vi "Auto_Routine_RightTwoPieceThen2CenterTRAJ.vi"   [LabVIEW 2023]
uses:
  Shoulder/ShoulderGetSetpointEnum.ctl
  Trajectory/TrajectoryGlobals.vi
  <vilib>/Rock Robotics/WPI/ThirdParty/JAS_Junk/TrajLib/Trajectory_Library.lvlib
types:
  T1 = typedef "ShoulderGetSetpointEnum.ctl" = enum16{"ShoulderRest", "ShoulderSpeaker", "ShoulderAmp"}
  T2 = typedef "ShoulderGetSetpointEnum.ctl" = enum16{"ShoulderRest", "ShoulderShoot", "ShoulderAmp", "ArmFloorPickup", "ArmAmpDeposit", "ArmSpeakerShoot", "ArmStartPosition", "ArmRestPosition", "ArmSourceIntake", "ArmAwayShoot"}
  T3 = typedef "Trajectory_Library.lvlib/TRAJECTORY.ctl" = cluster{"TotalTImeSecs":dbl, "States":T4[]}
  T4 = typedef "Trajectory_Library.lvlib/TRAJ_STATE.ctl" = cluster{"TimeSeconds":dbl, "Velocity":dbl, "Acceleration":dbl, "POSE":T5, "Curvature":dbl}
  T5 = typedef "Trajectory_Library.lvlib/POSE2D.ctl" = cluster{"TRANSLATION":T6, "ROTATION":T7}
  T6 = typedef "Trajectory_Library.lvlib/TRANSLATION2D.ctl" = cluster{"X":dbl, "Y":dbl}
  T7 = typedef "Trajectory_Library.lvlib/ROTATION2D.ctl" = cluster{"VALUE":dbl, "COS":dbl, "SIN":dbl}
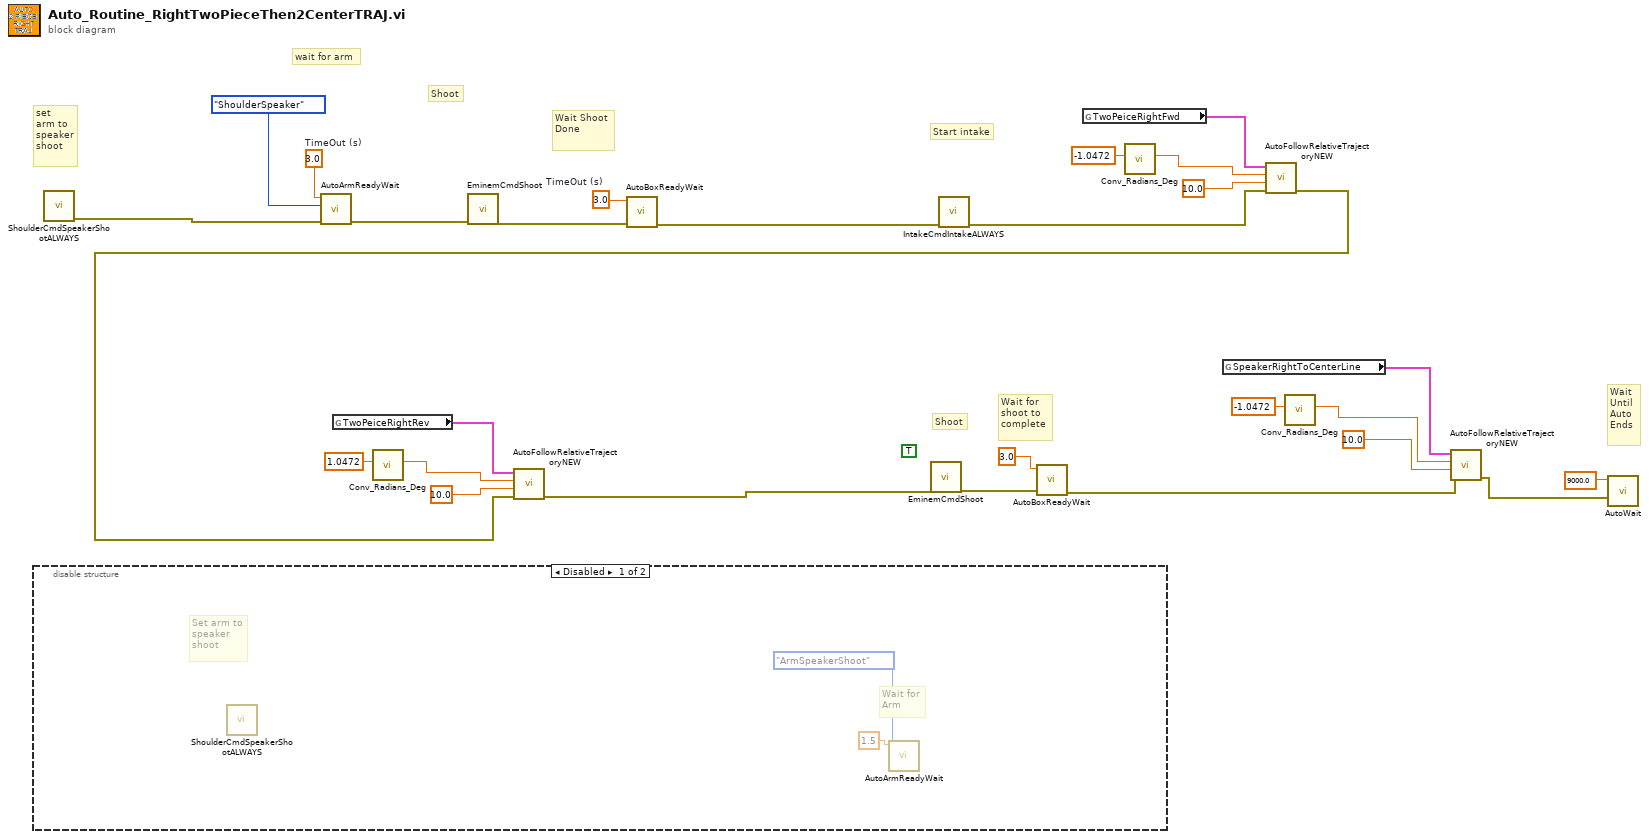
[diagram p0: block diagram]
diagram:
  (unwired) TRUE ("Box shoot")
  w27 = 3.0  # TimeOut (s)
  w24 = 3.0  # TimeOut (s)
  # "Wait\nUntil\nAuto \nEnds"
  # "Wait for\nshoot to\ncomplete"
  # "Shoot"
  # "Start intake"
  # "Wait Shoot\nDone"
  # "Shoot"
  # "set \narm to\nspeaker\nshoot"
  # "wait for arm"
  n1 = disable-structure shown="Disabled" {
    frame Disabled {
      # "Wait for\nArm"
      # "Set arm to\nspeaker \nshoot"
      n2 = call "ShoulderCmdSpeakerShootALWAYS.vi"() -> ()  [unwired: 11 in, 1 out]
      n3 = call "AutoArmReadyWait.vi"("ArmSetpoints"=ShoulderGetSetpointEnum."ArmSpeakerShoot", "TimeOut (s)"=1.5) -> ("error in (no error)"=w28:errorcluster)  [unwired: 8 in, 1 out]
    }
    frame Enabled {
    }
  }
  n4 = call "ShoulderCmdSpeakerShootALWAYS.vi"() -> ("error out"=w2:errorcluster)  [unwired: 11 in]
  n5 = call "AutoArmReadyWait.vi"("error in (no error)"=w2, "ArmSetpoints"=ShoulderGetSetpointEnum."ShoulderSpeaker", "TimeOut (s)"=w27) -> ("error out"=w25:errorcluster)  [unwired: 8 in]
  n6 = global read "TrajectoryGlobals.vi" "TwoPeiceRightRev"() -> (w16:T3)
  n7 = call <vilib>:"Conv_Radians_Deg.vi"("Radians"=1.0472) -> ("Degrees"=w14:dbl)  [unwired: 10 in]
  n8 = call "EminemCmdShoot.vi"("error in (no error)"=w25) -> ("error out"=w26:errorcluster)  [unwired: 10 in]
  n9 = call "AutoBoxReadyWait.vi"("error in (no error)"=w26, "TimeOut (s)"=w24) -> ("error out"=w4:errorcluster)  [unwired: 9 in]
  n10 = call "IntakeCmdIntakeALWAYS.vi"("error in (no error)"=w4) -> ("error out"=w3:errorcluster)  [unwired: 10 in]
  n11 = global read "TrajectoryGlobals.vi" "TwoPeiceRightFwd"() -> (w23:T3)
  n12 = call <vilib>:"Conv_Radians_Deg.vi"("Radians"=-1.0472) -> ("Degrees"=w21:dbl)  [unwired: 10 in]
  n13 = global read "TrajectoryGlobals.vi" "SpeakerRightToCenterLine"() -> (w12:T3)
  n14 = call "AutoFollowRelativeTrajectoryNEW.vi"("error in (no error)"=w3, "TimeOut (s)"=10.0, "End Orientation"=w21, "Trajectory"=w23) -> ("error out"=w6:errorcluster)  [unwired: 7 in]
  n15 = call "AutoFollowRelativeTrajectoryNEW.vi"("error in (no error)"=w6, "TimeOut (s)"=10.0, "End Orientation"=w14, "Trajectory"=w16) -> ("error out"=w1:errorcluster)  [unwired: 7 in]
  n16 = call "EminemCmdShoot.vi"("error in (no error)"=w1) -> ("error out"=w18:errorcluster)  [unwired: 10 in]
  n17 = call "AutoBoxReadyWait.vi"("error in (no error)"=w18, "TimeOut (s)"=3.0) -> ("error out"=w8:errorcluster)  [unwired: 9 in]
  n18 = call <vilib>:"Conv_Radians_Deg.vi"("Radians"=-1.0472) -> ("Degrees"=w10:dbl)  [unwired: 10 in]
  n19 = call "AutoFollowRelativeTrajectoryNEW.vi"("error in (no error)"=w8, "TimeOut (s)"=10.0, "End Orientation"=w10, "Trajectory"=w12) -> ("error out"=w7:errorcluster)  [unwired: 7 in]
  n20 = call "AutoWait.vi"("error in (no error)"=w7, "TimeOut (s)"=9000.0) -> ()  [unwired: 9 in, 1 out]
